vi "test_complement.vi"() -> ()   [LabVIEW 2018]
panel:
  out "Waveform Graph":dbl[][](graph)
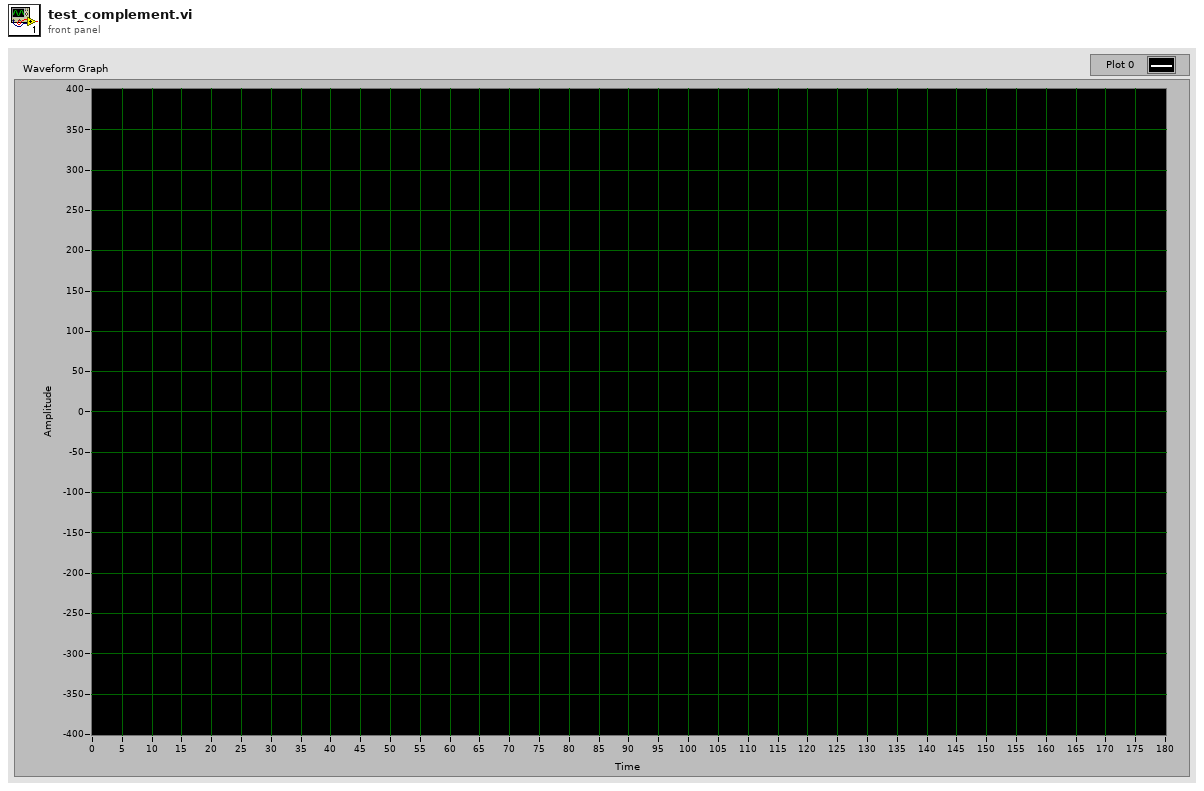
[diagram p1: front panel]
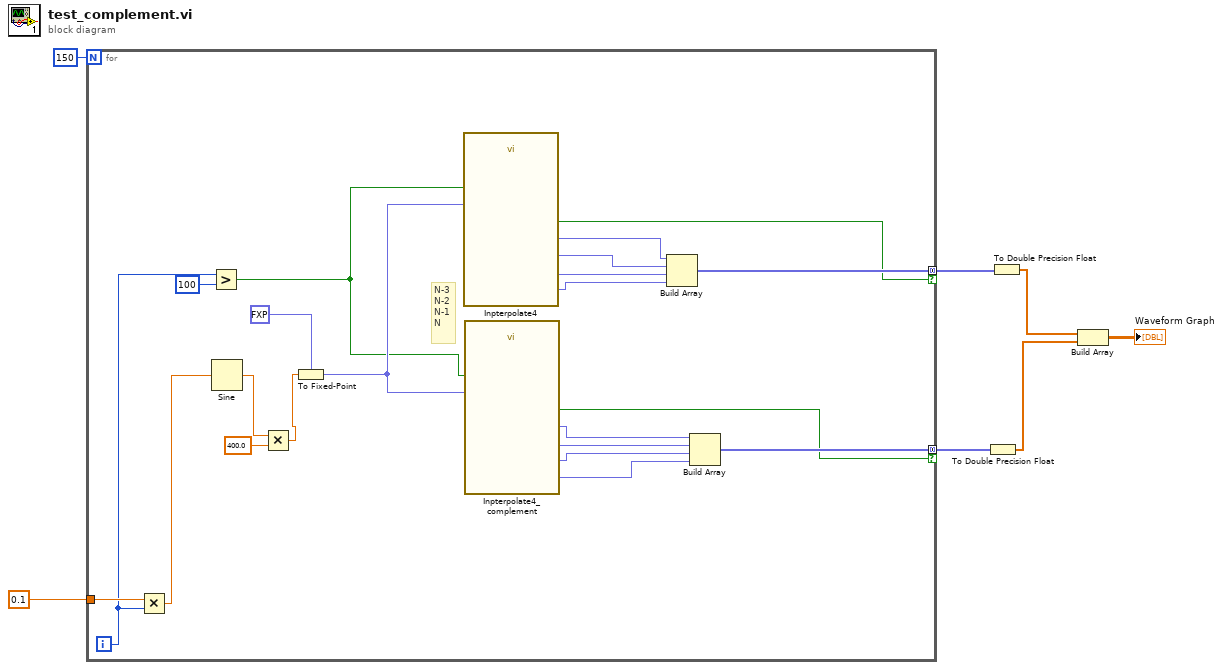
[diagram p0: block diagram]
diagram:
  n1 = for {
    N: 150 -> [_]
    tunnel: 0.1 -> [w29]
    tunnel: [w25] -> w6 mode=concatenating if=w24
    tunnel: [w23] -> w5 mode=concatenating if=w22
    i -> [w21]
    # "N-3\nN-2\nN-1\nN"
    n2 = Multiply(x=w29, y=w21) -> (x*y=w28:dbl)
    n3 = Greater?(x=w21, y=100) -> (0:w19:bool)
    n4 = Sine(x=w28) -> (sin(x)=w18:dbl)
    n5 = Multiply(x=w18, y=400.0) -> (x*y=w16:dbl)
    n6 = To Fixed-Point(fixed-point type=fxp<+/-,16,14> 0.0 ("X"), number=w16) -> (fixed-point=w26:fxp<+/-,16,14>)
    n7 = call "Inpterpolate4.vi"("X"=w26, "input valid"=w19) -> ("X(t)"=w15:fxp<+/-,16,14>, "X(t -1)"=w14:fxp<+/-,16,14>, "X(t -2)"=w13:fxp<+/-,16,14>, "X(t -3)"=w12:fxp<+/-,16,14>, "output valid"=w24:bool)  [unwired: 9 in]
    n8 = call "Inpterpolate4_complement.vi"("X"=w26, "input valid"=w19) -> ("X(t)"=w11:fxp<+/-,16,14>, "X(t -1)"=w10:fxp<+/-,16,14>, "X(t -2)"=w9:fxp<+/-,16,14>, "X(t -3)"=w8:fxp<+/-,16,14>, "output valid"=w22:bool)  [unwired: 9 in]
    n9 = Build Array(w12, w13, w14, w15) -> (w25:fxp<+/-,16,14>[])
    n10 = Build Array(w8, w9, w10, w11) -> (w23:fxp<+/-,16,14>[])
  }
  n11 = To Double Precision Float(number=w5) -> (double precision float=w3:dbl[])
  n12 = To Double Precision Float(number=w6) -> (double precision float=w4:dbl[])
  n13 = Build Array(w4, w3) -> (→"Waveform Graph":dbl[][])
